vi "Write Altitude.vi"(8 "error in (no error)":errorcluster, 10 "Altitude":dbl, 11 "Task Data in":refnum<class "Task Data.lvclass">) -> (0 "error out":errorcluster, 3 "Task Data out":refnum<class "Task Data.lvclass">)   [LabVIEW 2012, in "Task Data.lvclass"]
uses:
  Task Data.lvclass
  Task Data.lvclass/Task Data.ctl
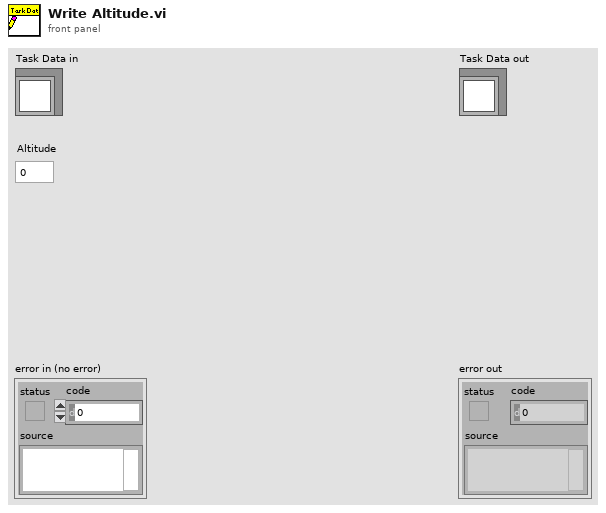
[diagram p1: front panel]
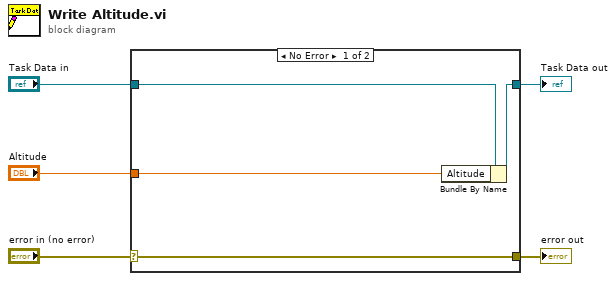
[diagram p0: block diagram]
diagram:
  n1 = case shown="No Error" "error in (no error)" {
    selector: "error in (no error)" -> [w9 w10]
    tunnel: [w9 w10] -> w4
    tunnel: [w7 w11] -> w2
    tunnel: "Task Data in" -> [w8 w11]
    tunnel: "Altitude" -> [w6 _]
    frame No Error {
      n2 = Bundle By Name(cluster=w8, "Altitude"=w6) -> (w7:refnum<class "Task Data.lvclass">)
    }
    frame Error {
    }
  }
  "error out" <- w4
  "Task Data out" <- w2
